vi "Lake Shore 335 Configure Output Control Parameters.vi"(0 "VISA resource name":refnum<visa-resource-name>="COM3") -> ()   [LabVIEW 2017]
doc: "This VI was designed to demonstrate typical usage of sub VIs containing the more common 335 functions. The VI Initializes the instrument, allows the user to determine if heater output control parameters and setpoint values are sent, takes a single sensor reading, and then closes the instrument."
uses:
  <instrlib>/Lake Shore 335/Public/Data/Sensor Data (Single Reading).vi
  <instrlib>/Lake Shore 335/Lake Shore 335.lvlib
panel:
  in  "Polarity (0:Unipolar)":u16(ring) items=["Unipolar", "Bipolar"]
  in  "Output Type (0:Current)":u16(ring) items=["Current", "Voltage"]
  in  "Heater Output (1:1)":u16(ring)=1 items=["1"=1, "2"=2]
  in  "Heater Resistance (1:25 Ohm)":u16(ring)=2 items=["25 Ohm"=1, "50 Ohm"=2]
  in  "Max User Current (1.732)":dbl=1.732 format="%.3f"
  in  "Heater Out Display (1:Current)":u16(ring)=1 items=["Current"=1, "Power"=2]
  in  "Max Current (0:User Specified)":u16(ring)=2 items=["User Specified", "0.707 A", "1.0 A", "1.141 A", "1.732 A"]
  in  "Mode (0:Off)":u16(ring)=1 items=["Off", "Closed Loop PID", "Zone", "Open Loop", "Monitor Out", "Warmup Supply"]
  in  "Power Up Enable (F: Off)":bool
  in  "Input (0:None)":u16(ring)=1 items=["None", "A", "B"]
  in  "Input (0:A)":u16(ring) items=["A", "B"]
  in  "Data Source (0:Kelvin)":u16(ring) items=["Kelvin", "Celsius", "Sensor Units"]
  out "Sensor Data":dbl=124.44 format="%.4f"
  in  "Configure Setpoint (0: Don't Configure)":u16(ring) items=["Don't Configure", "Configure"]
  in  "Setpoint (0.0000)":dbl format="%.4f"
  in  "Manual Output (0.00 %)":dbl format="%.2f"
  in  "Range (0:Off)":u16(ring)=1 items=["Off", "Low (On)", "Medium", "High"]
  in  "Rate (D) (0.0 %)":dbl format="%.1f"
  in  "Reset (I) (20.0)":dbl=20.0 format="%.1f"
  in  "Gain (P) (50.0)":dbl=50.0 format="%.1f"
  in  "Serial Configuration":T1={"Baud Rate"=57600, "Parity"=1, "Data Bits"=7, "Stop Bits"=10, "Flow Control"=0} {"Flow Control" items=["None", "XON/XOFF", "RTS/CTS", "XON/XOFF & RTS/CTS", "DTR/DSR", "XON/XOFF & DTR/DSR"]; "Stop Bits" items=["1.0"=10, "1.5"=15, "2.0"=20]; "Data Bits" items=["7"=7, "8"=8]; "Parity" items=["None", "Odd", "Even", "Mark", "Space"]; "Baud Rate" items=["300"=300, "600"=600, "1200"=1200, "2400"=2400, "4800"=4800, "9600"=9600, "19200"=19200, "38400"=38400, "57600"=57600]}
  in  "Configure Control Parameters (0: Don't Configure)":u16(ring)=1 items=["Don't Configure", "Configure"]
  # "(c) 2011 Lake Shore Cryotronics Inc.  ALL RIGHTS RESERVED."
  # "(c) 2020 SIE.SAI MODIFICADO.  ALL RIGHTS RESERVED."
  # "Output Control Parameters"
  # "Output Setpoint"
  # "Settings for Either Heater Output"
  # "Sensor Data"
  # "Settings for Heater Output 2 Only"
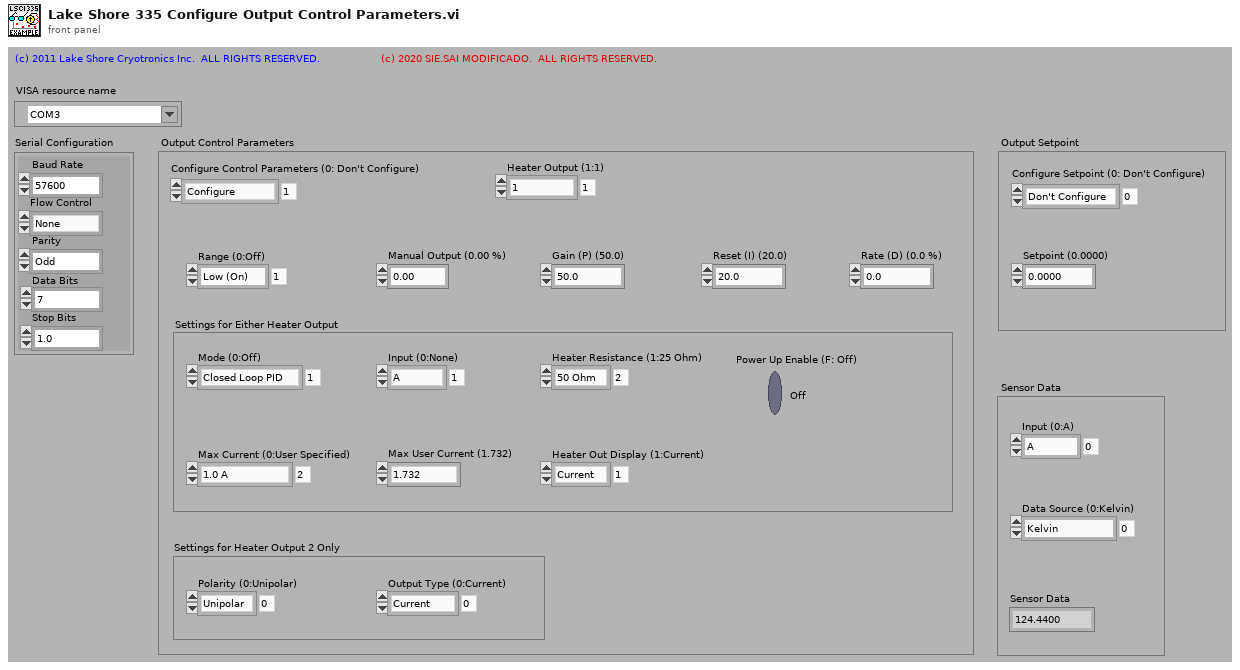
[diagram p1: front panel]
types:
  T1 = cluster{"Baud Rate":u32, "Parity":u16, "Data Bits":u16, "Stop Bits":u16, "Flow Control":u16}
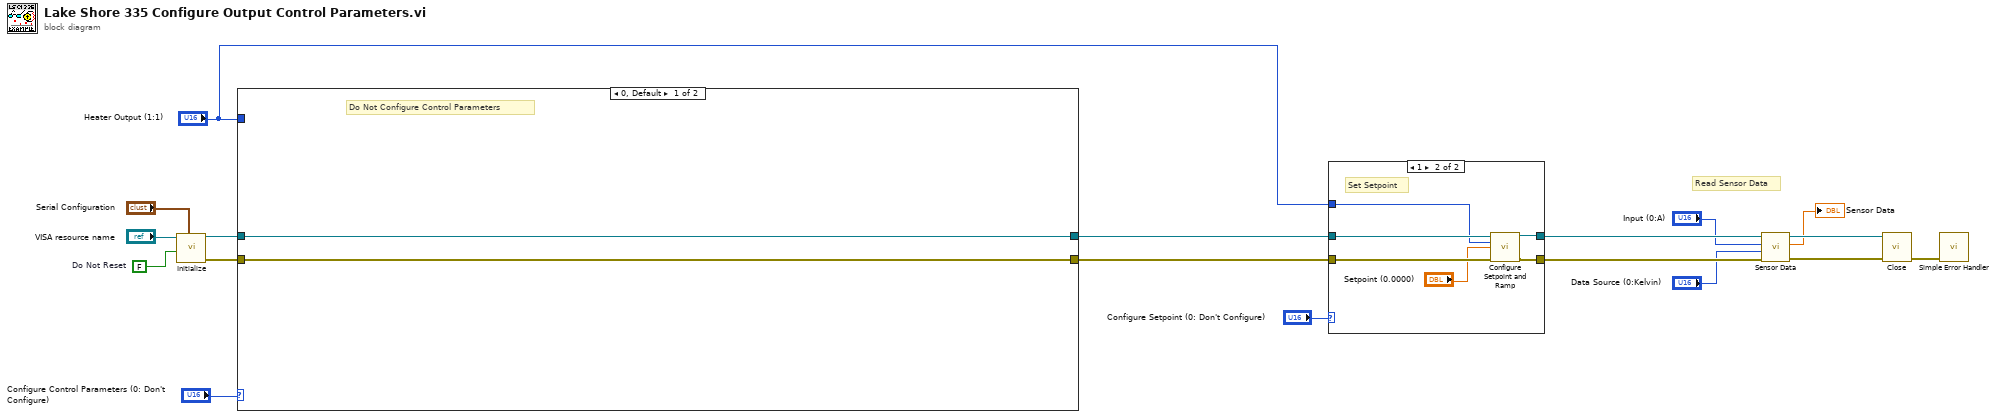
[diagram p0: block diagram]
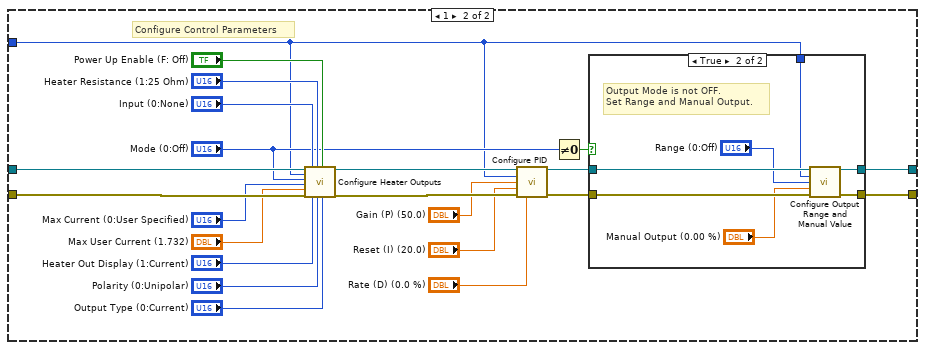
[diagram p3: hidden frame]
diagram:
  w11 = FALSE  # Do Not Reset
  # "Read Sensor Data"
  n1 = call <instrlib>:"Initialize.vi"("Serial Configuration"="Serial Configuration", "Reset (True)"=w11, "VISA resource name"="VISA resource name") -> ("error out"=w17:errorcluster, "VISA resource name out"=w18:refnum<visa-resource-name>)  [unwired: 7 in]
  n2 = case shown="0, Default" "Configure Control Parameters (0: Don't Configure)" {
    tunnel: "Heater Output (1:1)" -> [_ w21]
    tunnel: w18 -> [w20 w36]
    tunnel: w17 -> [w19 w35]
    tunnel: [w19 w40] -> w12
    tunnel: [w20 w39] -> w13
    frame 0, Default {
      # "Do Not Configure Control Parameters"
    }
    frame 1 {
      # "Configure Control Parameters"
      n3 = call <instrlib>:"Configure Heater Outputs.vi"("VISA resource name"=w36, "Heater Output (1:1)"=w21, "Mode (0:Off)"="Mode (0:Off)", "Max Current (0:User Specified)"="Max Current (0:User Specified)", "Max User Current (1.732)"="Max User Current (1.732)", "error in (no error)"=w35, "Input (0:None)"="Input (0:None)", "Heater Out Display (1:Current)"="Heater Out Display (1:Current)", "Heater Resistance (1:25 Ohm)"="Heater Resistance (1:25 Ohm)", "Polarity (0:Unipolar)"="Polarity (0:Unipolar)", "Power Up Enable (F: Off)"="Power Up Enable (F: Off)", "Output Type (0:Current)"="Output Type (0:Current)") -> ("VISA resource name out"=w38:refnum<visa-resource-name>, "error out"=w37:errorcluster)  [unwired: 6 in]
      n4 = call <instrlib>:"Configure PID.vi"("VISA resource name"=w38, "Output's Control Loop (1:1)"=w21, "Gain (P) (50.0)"="Gain (P) (50.0)", "Reset (I) (20.0)"="Reset (I) (20.0)", "error in (no error)"=w37, "Rate (D) (0.0 %)"="Rate (D) (0.0 %)") -> ("VISA resource name out"=w42:refnum<visa-resource-name>, "error out"=w41:errorcluster)  [unwired: 8 in]
      n5 = Not Equal To 0?(x="Mode (0:Off)") -> (x != 0?=w31:bool)
      n6 = case shown="True" w31 {
        tunnel: w42 -> [w44 w51]
        tunnel: w41 -> [w43 w50]
        tunnel: [w43 w49] -> w40
        tunnel: [w44 w48] -> w39
        tunnel: w21 -> [_ w47]
        frame False {
          # "Output Mode is OFF.  Do not\nset Range and Manual Output (prevents \nExecution Error)."
        }
        frame True {
          # "Output Mode is not OFF.\nSet Range and Manual Output."
          n7 = call <instrlib>:"Configure Output Range and Manual Value.vi"("VISA resource name"=w51, "Heater Output (1:1)"=w47, "Range (0:Off)"="Range (0:Off)", "Manual Output (0.00 %)"="Manual Output (0.00 %)", "error in (no error)"=w50) -> ("VISA resource name out"=w48:refnum<visa-resource-name>, "error out"=w49:errorcluster)  [unwired: 9 in]
        }
      }
    }
  }
  n8 = case shown="1" "Configure Setpoint (0: Don't Configure)" {
    tunnel: "Heater Output (1:1)" -> [_ w57]
    tunnel: w13 -> [w53 w58]
    tunnel: w12 -> [w52 w59]
    tunnel: [w52 w55] -> w8
    tunnel: [w53 w56] -> w9
    frame 0, Default {
      # "Do Not Set Setpoint"
    }
    frame 1 {
      # "Set Setpoint"
      n9 = call <instrlib>:"Configure Setpoint and Ramp.vi"("VISA resource name"=w58, "Output's Control Loop (1:1)"=w57, "Setpoint (0.0000)"="Setpoint (0.0000)", "error in (no error)"=w59) -> ("VISA resource name out"=w56:refnum<visa-resource-name>, "error out"=w55:errorcluster)  [unwired: 10 in]
    }
  }
  n10 = call-poly <instrlib>:"Sensor Data.vi"("error in (no error)"=w8, "Data Source (0:Kelvin)"="Data Source (0:Kelvin)", "Input (0:A)"="Input (0:A)", "VISA resource name"=w9) -> ("error out"=w6:errorcluster, "Sensor Data"=→"Sensor Data":dbl, "VISA resource name out"=w7:refnum<visa-resource-name>)  [unwired: 5 in]
  n11 = call <instrlib>:"Close.vi"("error in (no error)"=w6, "VISA resource name"=w7) -> ("error out"=w14:errorcluster)  [unwired: 9 in]
  n12 = call <vilib>:"Simple Error Handler.vi"("error in (no error)"=w14) -> ()  [unwired: 4 in, 5 out]
